vi "SubVI Set FP Channel-Guard value.vi"(3 "Value":bool, 5 "Ch ID":i32, 7 "Slave ID":i32, 10 "error in (no error)":errorcluster, 11 "Slaves ref array":refnum<vi>[][](array[refnum])) -> (2 "error out":errorcluster)   [LabVIEW 2020, in "QuPMXdriver.lvlib"]
uses:
  QuPMXdriver.lvlib
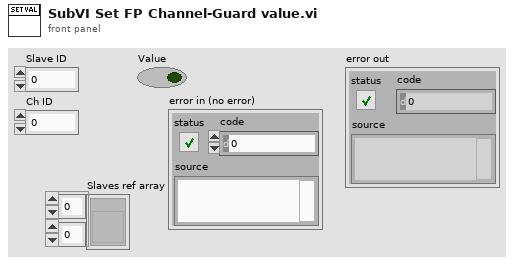
[diagram p1: front panel]
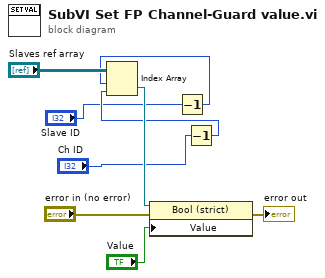
[diagram p0: block diagram]
diagram:
  n1 = Decrement(x="Slave ID") -> (x-1=w1:i32)
  n2 = Decrement(x="Ch ID") -> (x-1=w3:i32)
  n3 = Index Array(array="Slaves ref array", index (row)=w1, index (col)=w3) -> (element=w8:refnum<vi>)
  n4 = property class="Bool (strict)"(reference=w8, error in="error in (no error)", "Value"="Value") -> (error out=→"error out":errorcluster)  [unwired: 1 out]
